vi "image encryption.vi"() -> ()   [LabVIEW 2022 SP3]
uses:
  Row size.vi
  Column size.vi
  index values of B.vi
  index Values of G.vi
  index Values of R.vi
panel:
  in  "Original image Path":path=path "D:/Downloads chrome/parrot.jpg" caption="Image Path"
  out "Data values of B":dbl[](array[numeric])
  out "Data values of G":dbl[](array[numeric])
  out "Data values of R":dbl[](array[numeric])
  out "COVER IMAGE PIXMAP":u32[][](array[numeric]) format="%x"
  out "COVER IMAGE":picture
  in  "Cover  image Path":path
  out "DATA IMAGE PIXELS (U32)":u32[][](array[numeric])
  out "DATA IMAGE":T1(plugin-control)
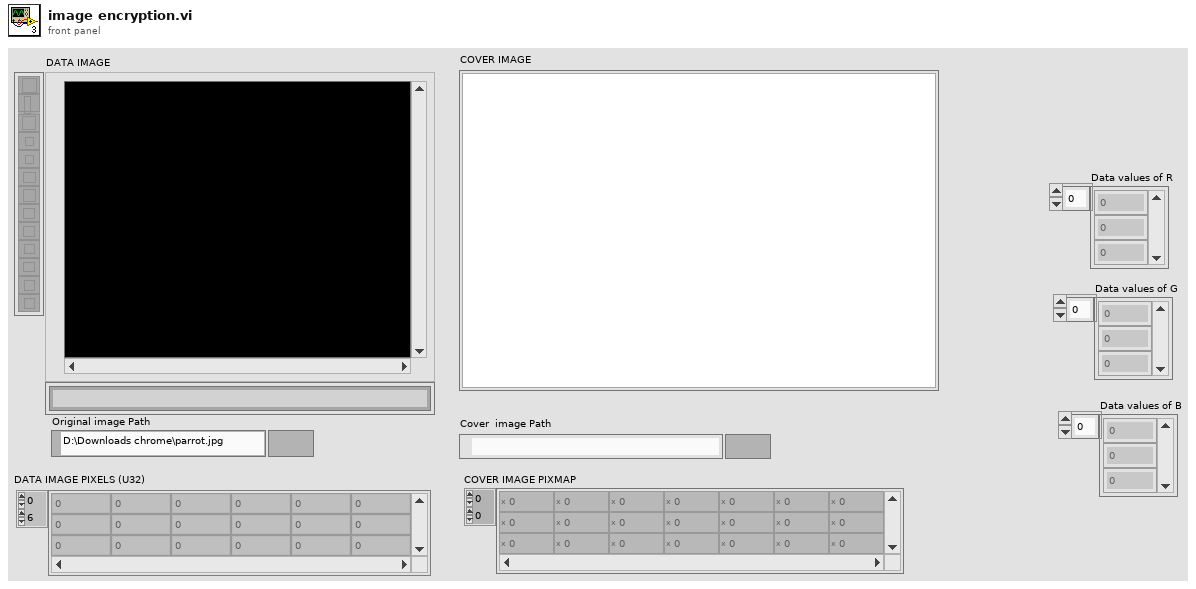
[diagram p1: front panel]
types:
  T1 = typedef "IMAQ Image.ctl" = refnum<image>
  T2 = typedef "imagedata.ctl" = cluster{"image type":i32, "image depth":i32, "image":u8[], "mask":u8[], "colors":u32[], "Rectangle":cluster{"left":i16, "top":i16, "right":i16, "bottom":i16}}
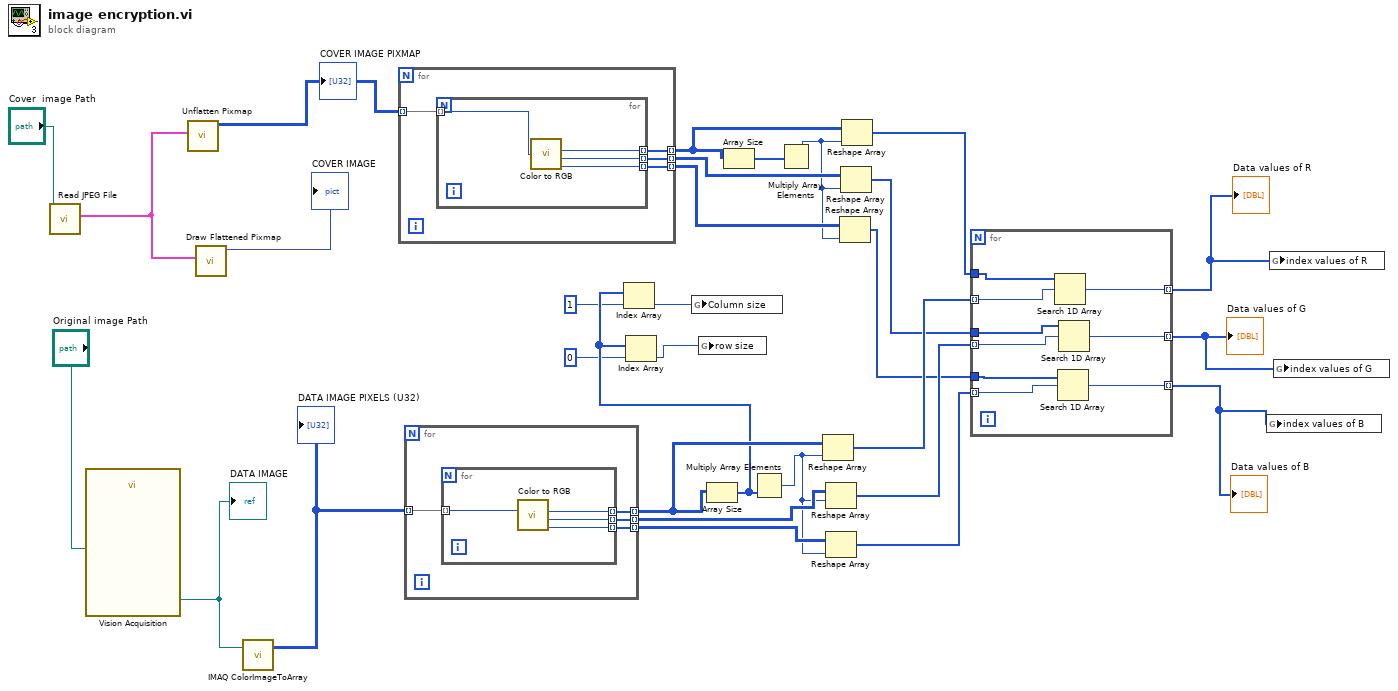
[diagram p0: block diagram]
diagram:
  n1 = call <vilib>:"Read JPEG File.vi"("path to JPEG file"="Cover  image Path") -> ("image data"=w23:T2)  [unwired: 8 in, 2 out]
  n2 = call "Vision Acquisition"("Image Path"="Original image Path") -> ("Image Out"=w30:T1)  [unwired: 25 in, 1 out]
  "DATA IMAGE" <- w30
  n3 = call <vilib>:"Unflatten Pixmap.vi"("image data"=w23) -> ("24-bit pixmap"=w16:u32[][])  [unwired: 4 in, 6 out]
  "COVER IMAGE PIXMAP" <- w16
  n4 = call <vilib>:"Draw Flattened Pixmap.vi"("image data"=w23) -> ("new picture"=→"COVER IMAGE":picture)  [unwired: 8 in]
  n5 = call "IMAQ ColorImageToArray"("Image"=w30) -> ("Image Pixels (U32)"=w29:u32[][])  [unwired: 3 in, 2 out]
  "DATA IMAGE PIXELS (U32)" <- w29
  n6 = for {
    tunnel: [w34] -> w20 mode=indexing
    tunnel: [w33] -> w22 mode=indexing
    tunnel: [w32] -> w21 mode=indexing
    tunnel: w16 -> [w31] mode=indexing
    n7 = for {
      tunnel: [w38] -> w34 mode=indexing
      tunnel: [w37] -> w33 mode=indexing
      tunnel: [w36] -> w32 mode=indexing
      tunnel: w31 -> [w35] mode=indexing
      n8 = call <vilib>:"Color to RGB.vi"("Color"=w35) -> ("R"=w38:u8, "G"=w37:u8, "B"=w36:u8)  [unwired: 1 out]
    }
  }
  n9 = for {
    tunnel: w29 -> [w42] mode=indexing
    tunnel: [w41] -> w28 mode=indexing
    tunnel: [w40] -> w27 mode=indexing
    tunnel: [w39] -> w26 mode=indexing
    n10 = for {
      tunnel: w42 -> [w46] mode=indexing
      tunnel: [w45] -> w41 mode=indexing
      tunnel: [w44] -> w40 mode=indexing
      tunnel: [w43] -> w39 mode=indexing
      n11 = call <vilib>:"Color to RGB.vi"("Color"=w46) -> ("R"=w45:u8, "G"=w44:u8, "B"=w43:u8)  [unwired: 1 out]
    }
  }
  n12 = Array Size(array=w28) -> (size(s)=w15:i32[])
  n13 = Index Array "Index Array"(array=w15, index=1) -> (element=w3:i32)
  n14 = Index Array(array=w15, index=0) -> (element=w2:i32)
  n15 = global write "Column size.vi" "Column size"(w3) -> ()
  n16 = global write "Row size.vi" "row size"(w2) -> ()
  n17 = Array Size(array=w20) -> (size(s)=w19:i32[])
  n18 = Multiply Array Elements(1:w15) -> (0:w18:i32)
  n19 = Multiply Array Elements(1:w19) -> (0:w17:i32)
  n20 = Reshape Array(w28, w18) -> (w12:u8[])
  n21 = Reshape Array(w27, w18) -> (w11:u8[])
  n22 = Reshape Array(w26, w18) -> (w10:u8[])
  n23 = Reshape Array(w21, w17) -> (w7:u8[])
  n24 = Reshape Array(w22, w17) -> (w8:u8[])
  n25 = Reshape Array "Reshape Array"(w20, w17) -> (w9:u8[])
  n26 = for {
    tunnel: w12 -> [w47] mode=indexing
    tunnel: w11 -> [w55] mode=indexing
    tunnel: w10 -> [w54] mode=indexing
    tunnel: w9 -> [w53]
    tunnel: w8 -> [w52]
    tunnel: w7 -> [w51]
    tunnel: [w50] -> w6 mode=indexing
    tunnel: [w49] -> w5 mode=indexing
    tunnel: [w48] -> w4 mode=indexing
    n27 = Search 1D Array(1D array=w53, element=w47) -> (index of element=w50:i32)  [unwired: 1 in]
    n28 = Search 1D Array(1D array=w51, element=w54) -> (index of element=w48:i32)  [unwired: 1 in]
    n29 = Search 1D Array(1D array=w52, element=w55) -> (index of element=w49:i32)  [unwired: 1 in]
  }
  "Data values of R" <- w6
  "Data values of G" <- w5
  "Data values of B" <- w4
  n30 = global write "index values of B.vi" "index values of B"(w4) -> ()
  n31 = global write "index Values of R.vi" "index values of R"(w6) -> ()
  n32 = global write "index Values of G.vi" "index values of G"(w5) -> ()
